vi "Stoplight.vi"() -> ()   [LabVIEW 2023]
uses:
  <vilib>/numeric/Random Number (Range) U64.vi
  <vilib>/numeric/sub_Random U32.vi
panel:
  out "EV Img C":dbl(slide) scale=0.0..10.0
  out "EV img A":dbl(slide) scale=0.0..10.0
  out "EV img b":dbl(slide) scale=0.0..10.0
  out "Car img  C":dbl(slide) scale=0.0..10.0
  out "Car img A":dbl(slide) scale=0.0..10.0
  out "Car img B":dbl(slide) scale=0.0..10.0
  out "EV Alert":bool
  out "EV Changer":dbl
  out "Emergency Lane":bool
  out "stopper":bool
  out "Numeric":i32
  out "EV Num":dbl
  out "Timer":dbl
  in  "Next Lane":string
  out "Indicator":dbl
  in  "Add EV  C":bool
  in  "Add EV  B":bool
  in  "Add EV  A":bool
  in  "Add Ped  C":bool
  in  "Add Ped  B":bool
  in  "Add  Ped A":bool
  in  "Add Car C":bool
  in  "Add Car  B":bool
  in  "Add Car A":bool
  out "Emergency Vehicle C":bool
  out "Emergency Vehicle B":bool
  out "Emergency Vehicle A":bool
  out "Pedestrian C":dbl
  out "Pedestrian B":dbl
  out "Pedestrian A":dbl
  out "Cars C":dbl
  out "Cars B":dbl
  out "Cars A":dbl
  in  "stop":bool
  out "Lane 1g":bool
  out "Lane 3r":bool
  out "Lane 3y":bool
  out "Lane 3g":bool
  out "Lane 2r":bool
  out "Lane 2y":bool
  out "Lane 2g":bool
  out "Lane 1r":bool
  out "Lane 1y":bool
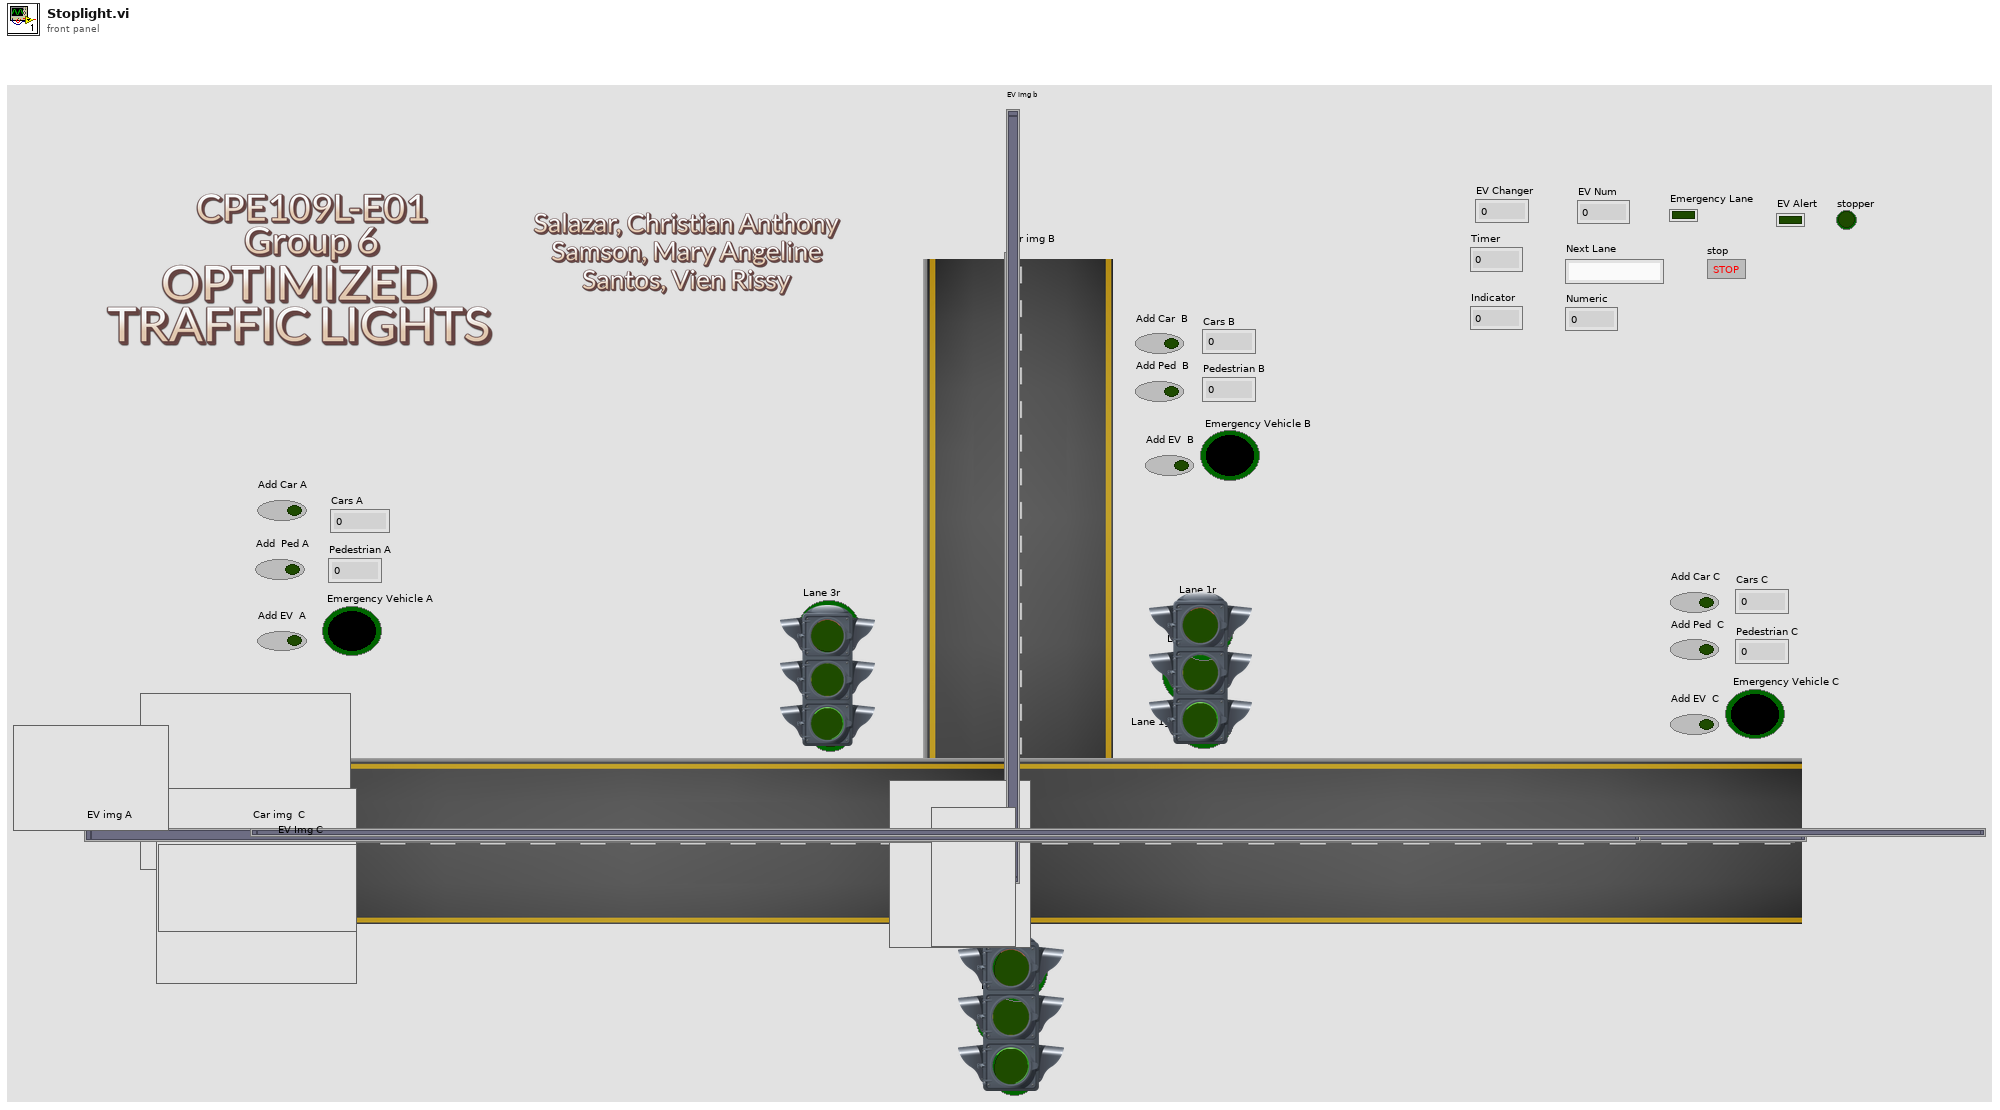
[diagram p1: front panel]
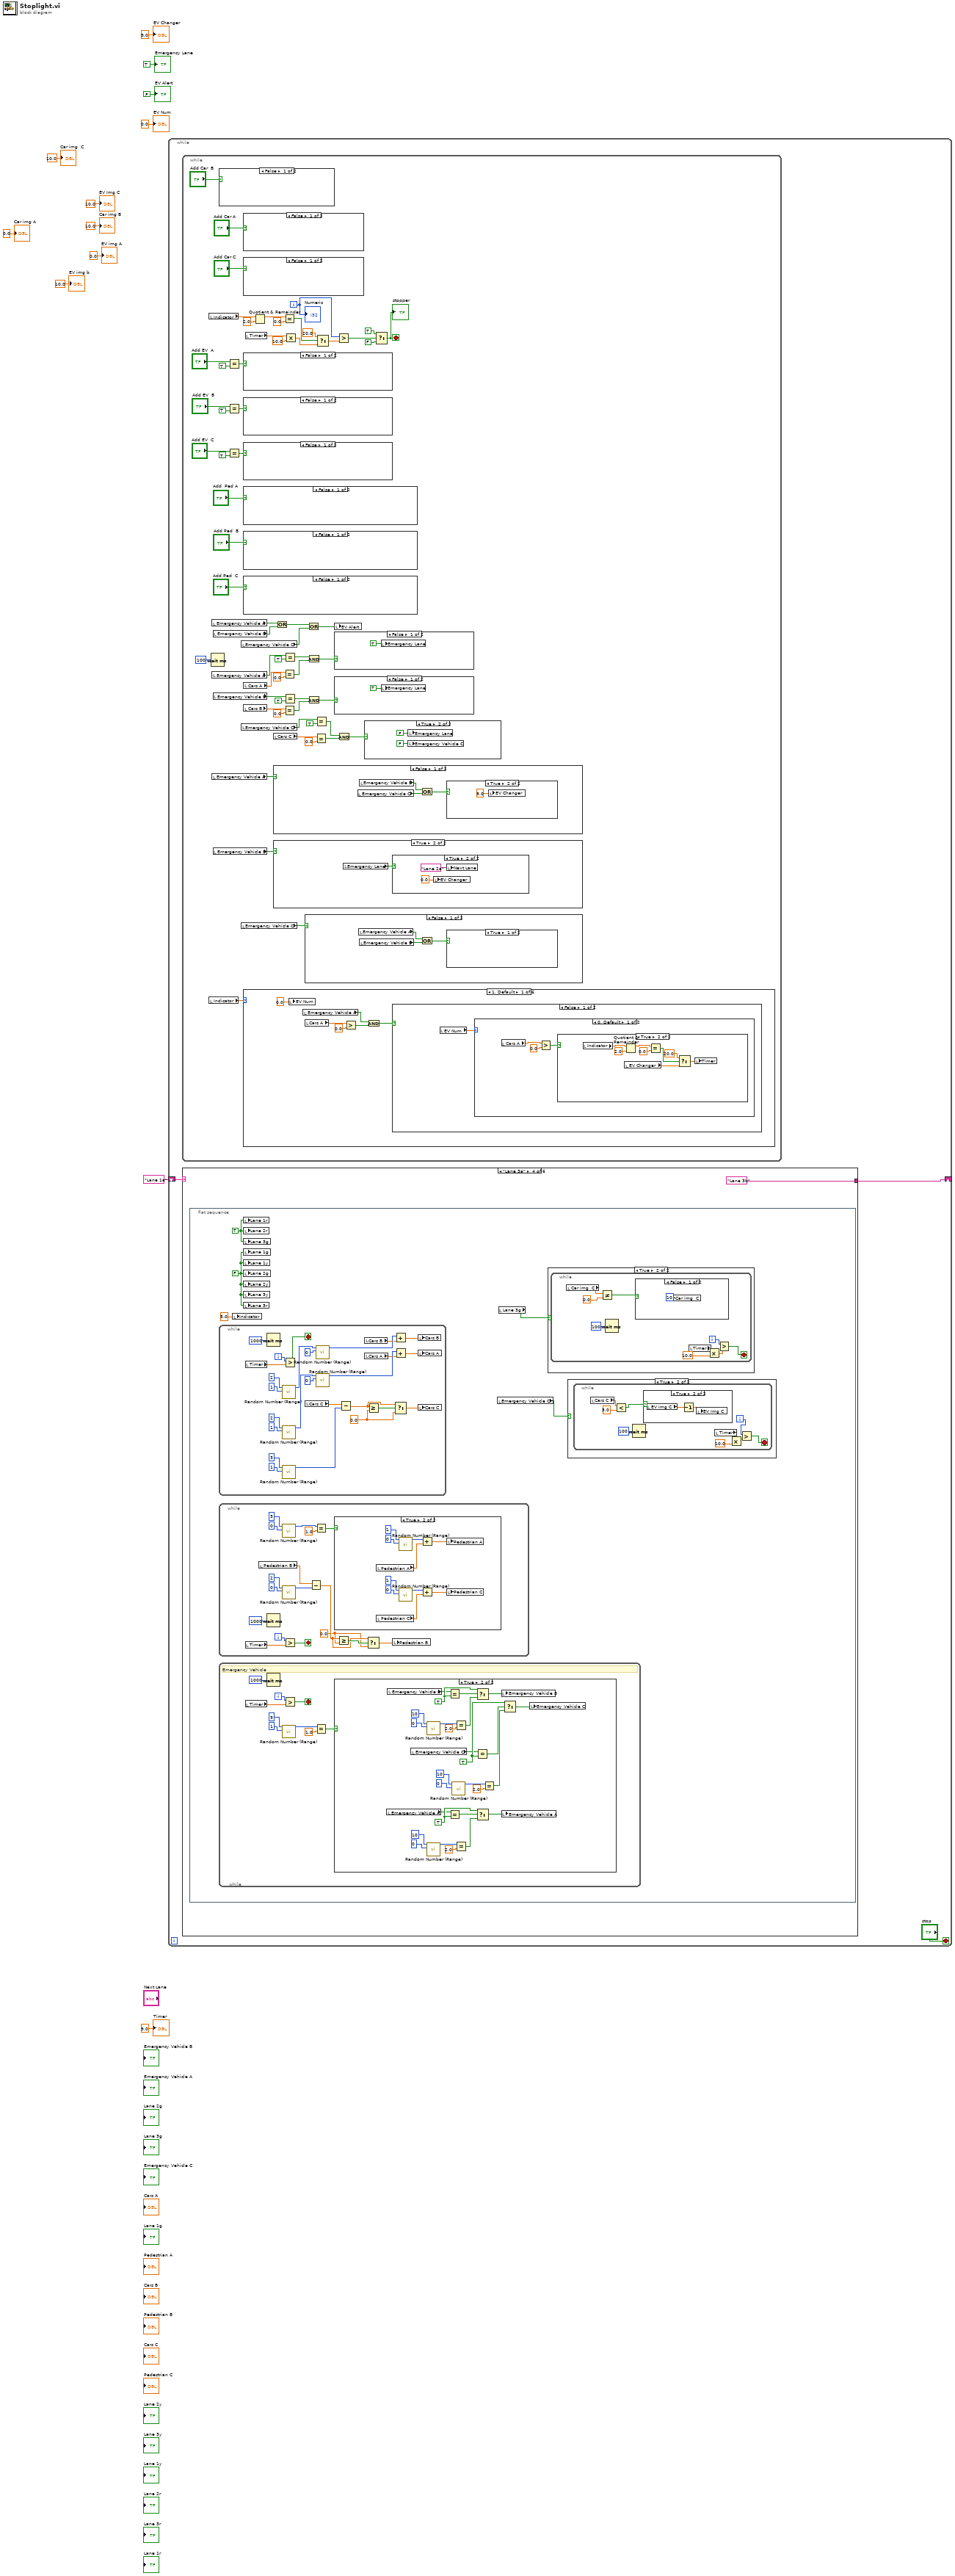
[diagram p0: block diagram]
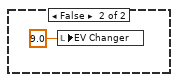
[diagram p2: hidden frame]
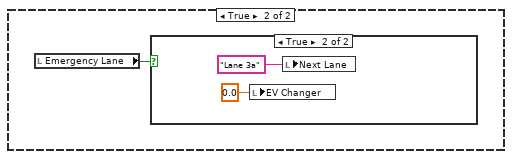
[diagram p3: hidden frame]
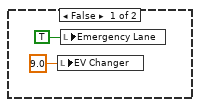
[diagram p4: hidden frame]
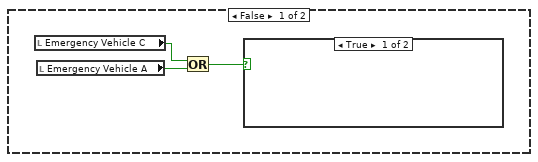
[diagram p5: hidden frame]
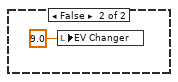
[diagram p6: hidden frame]
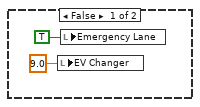
[diagram p7: hidden frame]
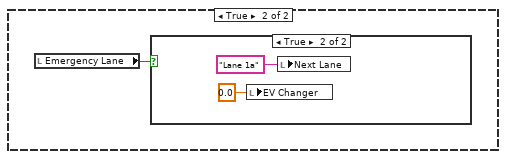
[diagram p9: hidden frame]
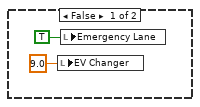
[diagram p10: hidden frame]
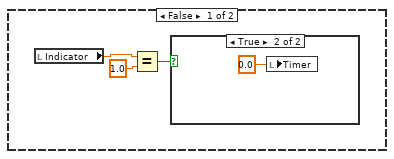
[diagram p11: hidden frame]
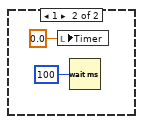
[diagram p13: hidden frame]
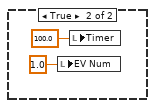
[diagram p14: hidden frame]
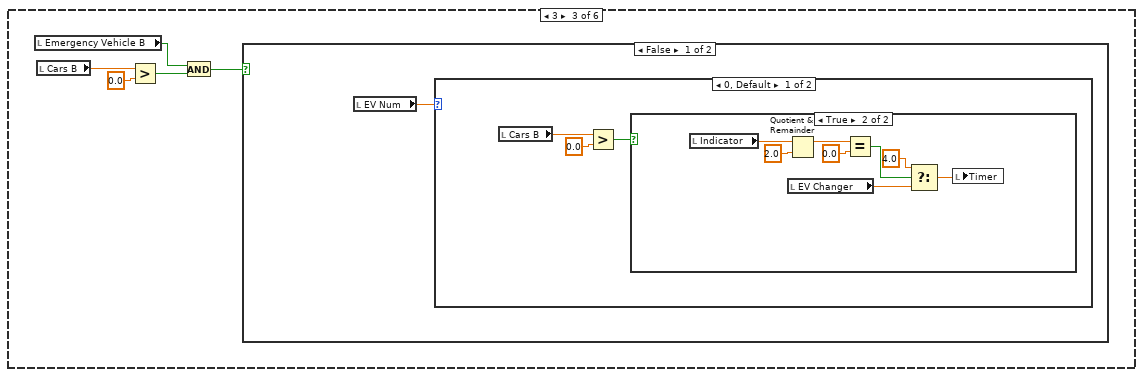
[diagram p16: hidden frame]
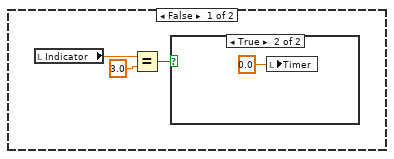
[diagram p17: hidden frame]
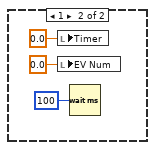
[diagram p19: hidden frame]
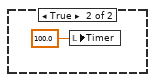
[diagram p20: hidden frame]
diagram:
  n1 = while {
    shift-right: [w13] -> _
    shift-left: "Lane 1a" -> [w14]
    stop <- "stop" stop-if-true
    n2 = while {
      i -> [w34]
      stop <- w73 stop-if-true
      n3 = local read "Indicator"() -> (w58:dbl)
      n4 = local read "Indicator"() -> (w39:dbl)
      n5 = Wait (ms)(milliseconds to wait=u32 100) -> ()  [unwired: 1 out]
      n6 = local read "Emergency Vehicle A"() -> (w20:bool)
      n7 = local read "Emergency Vehicle A"() -> (w45:bool)
      n8 = local read "Emergency Vehicle A"() -> (w32:bool)
      n9 = local read "Emergency Vehicle B"() -> (w19:bool)
      n10 = local read "Emergency Vehicle B"() -> (w43:bool)
      n11 = local read "Emergency Vehicle B"() -> (w31:bool)
      n12 = case shown="False" "Add Car  B" {
        frame False {
        }
        frame True {
          n13 = local read "Cars B"() -> (w201:dbl)
          n14 = Increment(x=w201) -> (x+1=w200:dbl)
          n15 = local write "Cars B"(w200) -> ()
        }
      }
      n16 = Equal?(x="Add EV  A", y=TRUE) -> (x = y?=w61:bool)
      n17 = Equal?(x="Add EV  B", y=TRUE) -> (x = y?=w60:bool)
      n18 = Equal?(x="Add EV  C", y=TRUE) -> (x = y?=w59:bool)
      n19 = local read "Emergency Vehicle C"() -> (w18:bool)
      n20 = local read "Emergency Vehicle C"() -> (w41:bool)
      n21 = local read "Emergency Vehicle C"() -> (w30:bool)
      n22 = case shown="False" "Add Car A" {
        frame False {
        }
        frame True {
          n23 = local read "Cars A"() -> (w203:dbl)
          n24 = Increment(x=w203) -> (x+1=w202:dbl)
          n25 = local write "Cars A"(w202) -> ()
        }
      }
      n26 = case shown="False" "Add Car C" {
        frame False {
        }
        frame True {
          n27 = local read "Cars C"() -> (w199:dbl)
          n28 = Increment(x=w199) -> (x+1=w198:dbl)
          n29 = local write "Cars C"(w198) -> ()
        }
      }
      n30 = case shown="False" w61 {
        frame False {
        }
        frame True {
          n31 = local write "Emergency Vehicle A"(TRUE ("Emergency Vehicle A")) -> ()
        }
      }
      n32 = case shown="False" w60 {
        frame False {
        }
        frame True {
          n33 = local write "Emergency Vehicle B"(TRUE ("Emergency Vehicle B")) -> ()
        }
      }
      n34 = case shown="False" w59 {
        frame False {
        }
        frame True {
          n35 = local write "Emergency Vehicle C"(TRUE ("Emergency Vehicle C")) -> ()
        }
      }
      n36 = case shown="False" "Add  Ped A" {
        frame False {
        }
        frame True {
          n37 = local read "Pedestrian A"() -> (w197:dbl)
          n38 = Increment(x=w197) -> (x+1=w196:dbl)
          n39 = local write "Pedestrian A"(w196) -> ()
        }
      }
      n40 = case shown="False" "Add Ped  B" {
        frame False {
        }
        frame True {
          n41 = local read "Pedestrian B"() -> (w195:dbl)
          n42 = Increment(x=w195) -> (x+1=w194:dbl)
          n43 = local write "Pedestrian B"(w194) -> ()
        }
      }
      n44 = case shown="False" "Add Ped  C" {
        frame False {
        }
        frame True {
          n45 = local read "Pedestrian C"() -> (w193:dbl)
          n46 = Increment(x=w193) -> (x+1=w192:dbl)
          n47 = local write "Pedestrian C"(w192) -> ()
        }
      }
      n48 = local read "Cars A"() -> (w44:dbl)
      n49 = local read "Cars B"() -> (w42:dbl)
      n50 = case shown="1, Default" w39 {
        frame 1, Default {
          n51 = local write "EV Num"(0.0 ("EV Num")) -> ()
          n52 = local read "Emergency Vehicle A"() -> (w107:bool)
          n53 = local read "Cars A"() -> (w108:dbl)
          n54 = Greater?(x=w108, y=0.0) -> (0:w106:bool)
          n55 = And(x=w107, y=w106) -> (x .and. y?=w105:bool)
          n56 = case shown="False" w105 {
            frame False {
              n57 = local read "EV Num"() -> (w110:dbl)
              n58 = case shown="0, Default" w110 {
                frame 0, Default {
                  n59 = local read "Cars A"() -> (w112:dbl)
                  n60 = Greater?(x=w112, y=0.0) -> (0:w113:bool)
                  n61 = case shown="True" w113 {
                    frame False {
                      n62 = local read "Indicator"() -> (w115:dbl)
                      n63 = Equal?(x=w115, y=1.0) -> (x = y?=w114:bool)
                      n64 = case shown="True" w114 {
                        frame False {
                        }
                        frame True {
                          n65 = local write "Timer"(0.0 ("Timer")) -> ()
                        }
                      }
                    }
                    frame True {
                      n66 = local read "Indicator"() -> (w119:dbl)
                      n67 = Quotient & Remainder(x=w119, y=2.0) -> (x-y*floor(x/y)=w123:dbl)  [unwired: 1 out]
                      n68 = local read "EV Changer"() -> (w118:dbl)
                      n69 = Equal?(x=w123, y=0.0) -> (x = y?=w124:bool)
                      n70 = Select(t=20.0, s=w124, f=w118) -> (s? t:f=w120:dbl)
                      n71 = local write "Timer"(w120) -> ()
                    }
                  }
                }
                frame 1 {
                  n72 = local write "Timer"(0.0) -> ()
                  n73 = Wait (ms)(milliseconds to wait=u32 100) -> ()  [unwired: 1 out]
                }
              }
            }
            frame True {
              n74 = local write "EV Num"(1.0 ("EV Num")) -> ()
              n75 = local write "Timer"(100.0) -> ()
            }
          }
        }
        frame 2 {
        }
        frame 3 {
          n76 = local read "Emergency Vehicle B"() -> (w132:bool)
          n77 = local read "Cars B"() -> (w133:dbl)
          n78 = Greater?(x=w133, y=0.0) -> (0:w131:bool)
          n79 = And(x=w132, y=w131) -> (x .and. y?=w130:bool)
          n80 = case shown="False" w130 {
            frame False {
              n81 = local read "EV Num"() -> (w135:dbl)
              n82 = case shown="0, Default" w135 {
                frame 0, Default {
                  n83 = local read "Cars B"() -> (w136:dbl)
                  n84 = Greater?(x=w136, y=0.0) -> (0:w138:bool)
                  n85 = case shown="True" w138 {
                    frame False {
                      n86 = local read "Indicator"() -> (w140:dbl)
                      n87 = Equal?(x=w140, y=3.0) -> (x = y?=w139:bool)
                      n88 = case shown="True" w139 {
                        frame False {
                        }
                        frame True {
                          n89 = local write "Timer"(0.0 ("Timer")) -> ()
                        }
                      }
                    }
                    frame True {
                      n90 = local read "Indicator"() -> (w144:dbl)
                      n91 = Quotient & Remainder(x=w144, y=2.0) -> (x-y*floor(x/y)=w148:dbl)  [unwired: 1 out]
                      n92 = local read "EV Changer"() -> (w143:dbl)
                      n93 = Equal?(x=w148, y=0.0) -> (x = y?=w149:bool)
                      n94 = Select(t=4.0, s=w149, f=w143) -> (s? t:f=w145:dbl)
                      n95 = local write "Timer"(w145) -> ()
                    }
                  }
                }
                frame 1 {
                  n96 = local write "Timer"(0.0) -> ()
                  n97 = local write "EV Num"(0.0) -> ()
                  n98 = Wait (ms)(milliseconds to wait=u32 100) -> ()  [unwired: 1 out]
                }
              }
            }
            frame True {
              n99 = local write "Timer"(100.0) -> ()
            }
          }
        }
        frame 4 {
        }
        frame 5 {
          n100 = local read "Emergency Vehicle C"() -> (w157:bool)
          n101 = local read "Cars C"() -> (w158:dbl)
          n102 = Greater?(x=w158, y=0.0) -> (0:w156:bool)
          n103 = And(x=w157, y=w156) -> (x .and. y?=w155:bool)
          n104 = case shown="False" w155 {
            frame False {
              n105 = local read "EV Num"() -> (w160:dbl)
              n106 = case shown="0, Default" w160 {
                frame 0, Default {
                  n107 = local read "Cars C"() -> (w162:dbl)
                  n108 = Greater?(x=w162, y=0.0) -> (0:w161:bool)
                  n109 = case shown="True" w161 {
                    frame False {
                      n110 = local read "Indicator"() -> (w165:dbl)
                      n111 = Equal?(x=w165, y=5.0) -> (x = y?=w164:bool)
                      n112 = case shown="False" w164 {
                        frame False {
                        }
                        frame True {
                          n113 = local write "Timer"(0.0 ("Timer")) -> ()
                        }
                      }
                    }
                    frame True {
                      n114 = local read "Indicator"() -> (w169:dbl)
                      n115 = Quotient & Remainder(x=w169, y=2.0) -> (x-y*floor(x/y)=w173:dbl)  [unwired: 1 out]
                      n116 = local read "EV Changer"() -> (w168:dbl)
                      n117 = Equal?(x=w173, y=0.0) -> (x = y?=w174:bool)
                      n118 = Select(t=4.0, s=w174, f=w168) -> (s? t:f=w170:dbl)
                      n119 = local write "Timer"(w170) -> ()
                    }
                  }
                }
                frame 1 {
                  n120 = local write "EV Num"(0.0) -> ()
                  n121 = local write "Timer"(0.0) -> ()
                  n122 = Wait (ms)(milliseconds to wait=u32 100) -> ()  [unwired: 1 out]
                }
              }
            }
            frame True {
              n123 = local write "Timer"(100.0) -> ()
            }
          }
        }
        frame 6 {
        }
      }
      n124 = local read "Timer"() -> (w37:dbl)
      n125 = Quotient & Remainder(x=w58, y=2.0) -> (x-y*floor(x/y)=w55:dbl)  [unwired: 1 out]
      n126 = local read "Cars C"() -> (w40:dbl)
      n127 = case shown="False" w32 {
        frame False {
          n128 = local read "Emergency Vehicle C"() -> (w96:bool)
          n129 = local read "Emergency Vehicle B"() -> (w97:bool)
          n130 = Or(x=w97, y=w96) -> (x .or. y?=w95:bool)
          n131 = case shown="True" w95 {
            frame False {
            }
            frame True {
              n132 = local write "EV Changer"(9.0 ("EV Changer")) -> ()
            }
          }
        }
        frame True {
          n133 = local read "Emergency Lane"() -> (w99:bool)
          n134 = case shown="True" w99 {
            frame False {
              n135 = local write "EV Changer"(9.0 ("EV Changer")) -> ()
              n136 = local write "Emergency Lane"(TRUE ("Emergency Lane")) -> ()
            }
            frame True {
              n137 = local write "EV Changer"(0.0 ("Timer")) -> ()
              n138 = local write "Next Lane"("Lane 1a" ("Next Lane")) -> ()
            }
          }
        }
      }
      n139 = case shown="True" w31 {
        frame False {
          n140 = local read "Emergency Vehicle C"() -> (w88:bool)
          n141 = local read "Emergency Vehicle A"() -> (w87:bool)
          n142 = Or(x=w88, y=w87) -> (x .or. y?=w86:bool)
          n143 = case shown="True" w86 {
            frame True {
            }
            frame False {
              n144 = local write "EV Changer"(9.0 ("EV Changer")) -> ()
            }
          }
        }
        frame True {
          n145 = local read "Emergency Lane"() -> (w90:bool)
          n146 = case shown="True" w90 {
            frame False {
              n147 = local write "EV Changer"(9.0 ("EV Changer")) -> ()
              n148 = local write "Emergency Lane"(TRUE ("Emergency Lane")) -> ()
            }
            frame True {
              n149 = local write "EV Changer"(0.0 ("Timer")) -> ()
              n150 = local write "Next Lane"("Lane 2a" ("Next Lane")) -> ()
            }
          }
        }
      }
      n151 = Or(x=w20, y=w19) -> (x .or. y?=w17:bool)
      n152 = Equal?(x=w55, y=0.0) -> (x = y?=w56:bool)
      n153 = Equal?(x=w44, y=0.0) -> (x = y?=w28:bool)
      n154 = Equal?(x=w42, y=0.0) -> (x = y?=w25:bool)
      n155 = Equal?(x=w45, y=TRUE) -> (x = y?=w29:bool)
      n156 = Equal?(x=w43, y=TRUE) -> (x = y?=w26:bool)
      n157 = Multiply(x=w37, y=10.0) -> (x*y=w36:dbl)
      n158 = case shown="False" w30 {
        frame False {
          n159 = local read "Emergency Vehicle A"() -> (w79:bool)
          n160 = local read "Emergency Vehicle B"() -> (w78:bool)
          n161 = Or(x=w79, y=w78) -> (x .or. y?=w77:bool)
          n162 = case shown="True" w77 {
            frame True {
            }
            frame False {
              n163 = local write "EV Changer"(9.0 ("EV Changer")) -> ()
            }
          }
        }
        frame True {
          n164 = local read "Emergency Lane"() -> (w81:bool)
          n165 = case shown="True" w81 {
            frame False {
              n166 = local write "EV Changer"(9.0 ("EV Changer")) -> ()
              n167 = local write "Emergency Lane"(TRUE ("Emergency Lane")) -> ()
            }
            frame True {
              n168 = local write "EV Changer"(0.0 ("Timer")) -> ()
              n169 = local write "Next Lane"("Lane 3a" ("Next Lane")) -> ()
            }
          }
        }
      }
      n170 = Or(x=w17, y=w18) -> (x .or. y?=w16:bool)
      n171 = And(x=w29, y=w28) -> (x .and. y?=w27:bool)
      n172 = And(x=w26, y=w25) -> (x .and. y?=w24:bool)
      n173 = Equal?(x=w40, y=0.0) -> (x = y?=w22:bool)
      n174 = Equal?(x=w41, y=TRUE) -> (x = y?=w23:bool)
      n175 = Select(t=20.0, s=w56, f=w36) -> (s? t:f=w35:dbl)
      n176 = local write "EV Alert"(w16) -> ()
      n177 = case shown="False" w27 {
        frame False {
          n178 = local write "Emergency Lane"(TRUE ("Emergency Lane")) -> ()
        }
        frame True {
          n179 = local write "Emergency Lane"(FALSE) -> ()
          n180 = local write "Emergency Vehicle A"(FALSE) -> ()
        }
      }
      n181 = case shown="False" w24 {
        frame False {
          n182 = local write "Emergency Lane"(TRUE ("Emergency Lane")) -> ()
        }
        frame True {
          n183 = local write "Emergency Lane"(FALSE) -> ()
          n184 = local write "Emergency Vehicle B"(FALSE ("Emergency Vehicle B")) -> ()
        }
      }
      n185 = Greater?(x=w34, y=w35) -> (0:w33:bool)
      n186 = And(x=w23, y=w22) -> (x .and. y?=w21:bool)
      n187 = case shown="True" w21 {
        frame False {
          n188 = local write "Emergency Lane"(TRUE ("Emergency Lane")) -> ()
        }
        frame True {
          n189 = local write "Emergency Lane"(FALSE) -> ()
          n190 = local write "Emergency Vehicle C"(FALSE ("Emergency Vehicle C")) -> ()
        }
      }
      n191 = Select(t=TRUE, s=w33, f=FALSE) -> (s? t:f=w73:bool)
      "stopper" <- w73
      "Numeric" <- w34
    }
    n192 = case shown="\"Lane 3a\"" w14 {
      tunnel: [w207 "Lane 2b" w334 "Lane 3b" w470 "Lane 1b"] -> w13
      frame "Lane 1b" {
        n193 = flat-sequence {
          frame #0 {
            w217 = FALSE
            w218 = TRUE
            n194 = local write "Timer"(4.0 ("Timer")) -> ()
            n195 = local write "Indicator"(2.0 ("Indicator")) -> ()
            n196 = Wait (ms)(milliseconds to wait=u32 2000) -> ()  [unwired: 1 out]
            n197 = local write "Lane 1g"(w217) -> ()
            n198 = local write "Lane 1r"(w217) -> ()
            n199 = local write "Lane 2g"(w217) -> ()
            n200 = local write "Lane 2y"(w217) -> ()
            n201 = local write "Lane 3g"(w217) -> ()
            n202 = local write "Lane 3y"(w217) -> ()
            n203 = local write "Lane 1y"(w218) -> ()
            n204 = local write "Lane 2r"(w218) -> ()
            n205 = local write "Lane 3r"(w218) -> ()
            n206 = local write "Car img B"(10) -> ()
            n207 = local write "EV img A"(0) -> ()
            n208 = local write "Car img  C"(10) -> ()
            n209 = local write "EV Img C"(10) -> ()
            n210 = local write "EV img b"(10) -> ()
            n211 = local write "Car img A"(0) -> ()
          }
        }
        n212 = local read "Next Lane"() -> (w204:string)
        n213 = local read "EV Alert"() -> (w206:bool)
        n214 = Select(t=w204, s=w206, f="Lane 2a") -> (s? t:f=w207:string)
      }
      frame "Lane 2a" {
        n215 = flat-sequence {
          frame #0 {
            w223 = FALSE
            w224 = TRUE
            n216 = while {
              stop <- w310 stop-if-true
              w322 = 0.0 ("y")
              # "Cars"
              n217 = Wait (ms)(milliseconds to wait=u32 1000) -> ()  [unwired: 1 out]
              n218 = call-poly <vilib>:"Random Number (Range).vi"("lower bound (0)"=u64 1, "upper bound (100)"=u64 2) -> ("number"=w311:u64)  [unwired: 9 in]
              n219 = call-poly <vilib>:"Random Number (Range).vi"("lower bound (0)"=u64 1, "upper bound (100)"=u64 2) -> ("number"=w314:u64)  [unwired: 9 in]
              n220 = call-poly <vilib>:"Random Number (Range).vi"("lower bound (0)"=u64 1, "upper bound (100)"=u64 3) -> ("number"=w317:u64)  [unwired: 9 in]
              n221 = local read "Cars B"() -> (w321:dbl)
              n222 = call-poly <vilib>:"Random Number (Range).vi"("lower bound (0)"=u64 0, "upper bound (100)"=w311) -> ("number"=w326:u64)  [unwired: 9 in]
              n223 = call-poly <vilib>:"Random Number (Range).vi"("lower bound (0)"=u64 0, "upper bound (100)"=w314) -> ("number"=w328:u64)  [unwired: 9 in]
              n224 = Subtract(x=w321, y=w317) -> (x-y=w323:dbl)
              n225 = local read "Cars C"() -> (w329:dbl)
              n226 = local read "Cars A"() -> (w330:dbl)
              n227 = Greater Or Equal?(x=w323, y=w322) -> (x >= y?=w324:bool)
              n228 = Add(x=w326, y=w329) -> (x+y=w325:dbl)
              n229 = Add(x=w328, y=w330) -> (x+y=w327:dbl)
              n230 = Select(t=w323, s=w324, f=w322) -> (s? t:f=w320:dbl)
              n231 = local read "stopper"() -> (w310:bool)
              n232 = local write "Cars C"(w325) -> ()
              n233 = local write "Cars A"(w327) -> ()
              n234 = local write "Cars B"(w320) -> ()
            }
            n235 = while {
              stop <- w285 stop-if-true
              w290 = 0.0 ("y")
              # "Pedestrian"
              n236 = local read "Pedestrian A"() -> (w293:dbl)
              n237 = Wait (ms)(milliseconds to wait=u32 1000) -> ()  [unwired: 1 out]
              n238 = call-poly <vilib>:"Random Number (Range).vi"("lower bound (0)"=u64 0, "upper bound (100)"=u64 3) -> ("number"=w295:u64)  [unwired: 9 in]
              n239 = call-poly <vilib>:"Random Number (Range).vi"("lower bound (0)"=u64 0, "upper bound (100)"=u64 2) -> ("number"=w286:u64)  [unwired: 9 in]
              n240 = Subtract(x=w293, y=w286) -> (x-y=w291:dbl)
              n241 = Equal?(x=w295, y=1.0) -> (x = y?=w294:bool)
              n242 = case shown="False" w294 {
                frame False {
                }
                frame True {
                  n243 = local read "Pedestrian B"() -> (w303:dbl)
                  n244 = local read "Pedestrian C"() -> (w301:dbl)
                  n245 = call-poly <vilib>:"Random Number (Range).vi"("lower bound (0)"=u64 0, "upper bound (100)"=u64 1) -> ("number"=w305:u64)  [unwired: 9 in]
                  n246 = call-poly <vilib>:"Random Number (Range).vi"("lower bound (0)"=u64 0, "upper bound (100)"=u64 1) -> ("number"=w304:u64)  [unwired: 9 in]
                  n247 = Add(x=w305, y=w303) -> (x+y=w302:dbl)
                  n248 = Add(x=w304, y=w301) -> (x+y=w300:dbl)
                  n249 = local write "Pedestrian B"(w302) -> ()
                  n250 = local write "Pedestrian C"(w300) -> ()
                }
              }
              n251 = Greater Or Equal?(x=w291, y=w290) -> (x >= y?=w292:bool)
              n252 = Select(t=w291, s=w292, f=w290) -> (s? t:f=w289:dbl)
              n253 = local write "Pedestrian A"(w289) -> ()
              n254 = local read "stopper"() -> (w285:bool)
            }
            n255 = while {
              stop <- w251 stop-if-true
              # "Emergency Vehicle"
              n256 = Wait (ms)(milliseconds to wait=u32 1000) -> ()  [unwired: 1 out]
              n257 = call-poly <vilib>:"Random Number (Range).vi"("lower bound (0)"=u64 1, "upper bound (100)"=u64 25) -> ("number"=w252:u64)  [unwired: 9 in]
              n258 = Equal?(x=w252, y=1.0) -> (x = y?=w254:bool)
              n259 = case shown="False" w254 {
                frame False {
                }
                frame True {
                  w266 = TRUE
                  w265 = TRUE
                  w264 = TRUE
                  n260 = local read "Emergency Vehicle A"() -> (w260:bool)
                  n261 = local read "Emergency Vehicle B"() -> (w259:bool)
                  n262 = local read "Emergency Vehicle C"() -> (w258:bool)
                  n263 = call-poly <vilib>:"Random Number (Range).vi"("lower bound (0)"=u64 0, "upper bound (100)"=u64 10) -> ("number"=w274:u64)  [unwired: 9 in]
                  n264 = call-poly <vilib>:"Random Number (Range).vi"("lower bound (0)"=u64 0, "upper bound (100)"=u64 10) -> ("number"=w275:u64)  [unwired: 9 in]
                  n265 = Equal?(x=w259, y=w265) -> (x = y?=w268:bool)
                  n266 = Equal?(x=w260, y=w264) -> (x = y?=w269:bool)
                  n267 = call-poly <vilib>:"Random Number (Range).vi"("lower bound (0)"=u64 0, "upper bound (100)"=u64 10) -> ("number"=w273:u64)  [unwired: 9 in]
                  n268 = Equal?(x=w274, y=2.0) -> (x = y?=w262:bool)
                  n269 = Equal?(x=w275, y=2.0) -> (x = y?=w263:bool)
                  n270 = Select(t=w265, s=w268, f=w262) -> (s? t:f=w271:bool)
                  n271 = Equal?(x=w258, y=w266) -> (x = y?=w267:bool)
                  n272 = Select(t=w264, s=w269, f=w263) -> (s? t:f=w272:bool)
                  n273 = Equal?(x=w273, y=2.0) -> (x = y?=w261:bool)
                  n274 = local write "Emergency Vehicle B"(w271) -> ()
                  n275 = local write "Emergency Vehicle A"(w272) -> ()
                  n276 = Select(t=w266, s=w267, f=w261) -> (s? t:f=w270:bool)
                  n277 = local write "Emergency Vehicle C"(w270) -> ()
                }
              }
              n278 = local read "stopper"() -> (w251:bool)
            }
            n279 = local write "Indicator"(3.0 ("Indicator")) -> ()
            n280 = local write "Lane 1r"(w224) -> ()
            n281 = local write "Lane 2g"(w224) -> ()
            n282 = local write "Lane 3r"(w224) -> ()
            n283 = local write "Lane 1g"(w223) -> ()
            n284 = local write "Lane 1y"(w223) -> ()
            n285 = local write "Lane 2y"(w223) -> ()
            n286 = local write "Lane 2r"(w223) -> ()
            n287 = local write "Lane 3g"(w223) -> ()
            n288 = local write "Lane 3y"(w223) -> ()
            n289 = local read "Emergency Vehicle B"() -> (w220:bool)
            n290 = local read "Lane 2g"() -> (w221:bool)
            n291 = case shown="True" w221 {
              frame False {
                n292 = local write "Car img B"(10.0 ("Car img B")) -> ()
              }
              frame True {
                n293 = while {
                  i -> [w246]
                  stop <- w243 stop-if-true
                  n294 = local read "Car img B"() -> (w241:dbl)
                  n295 = Wait (ms)(milliseconds to wait=u32 100) -> ()  [unwired: 1 out]
                  n296 = Greater?(x=w241, y=1.0) -> (0:w239:bool)
                  n297 = case shown="True" w239 {
                    frame False {
                      n298 = local write "Car img B"(10.0 ("Car img B")) -> ()
                    }
                    frame True {
                      n299 = local read "Car img B"() -> (w250:dbl)
                      n300 = Decrement(x=w250) -> (x-1=w249:dbl)
                      n301 = local write "Car img B"(w249) -> ()
                    }
                  }
                  n302 = local read "Timer"() -> (w245:dbl)
                  n303 = Multiply(x=w245, y=10.0) -> (x*y=w242:dbl)
                  n304 = Greater?(x=w246, y=w242) -> (0:w243:bool)
                }
              }
            }
            n305 = case shown="True" w220 {
              frame False {
                n306 = local write "EV img b"(10.0 ("EV img b")) -> ()
              }
              frame True {
                n307 = while {
                  i -> [w229]
                  stop <- w227 stop-if-true
                  n308 = local read "Cars B"() -> (w233:dbl)
                  n309 = Less?(x=w233, y=5.0) -> (x < y?=w232:bool)
                  n310 = Wait (ms)(milliseconds to wait=u32 100) -> ()  [unwired: 1 out]
                  n311 = case shown="True" w232 {
                    frame False {
                      n312 = local write "EV img b"(10) -> ()
                    }
                    frame True {
                      n313 = local read "EV img b"() -> (w237:dbl)
                      n314 = Decrement(x=w237) -> (x-1=w236:dbl)
                      n315 = local write "EV img b"(w236) -> ()
                    }
                  }
                  n316 = local read "Timer"() -> (w231:dbl)
                  n317 = Multiply(x=w231, y=10.0) -> (x*y=w228:dbl)
                  n318 = Greater?(x=w229, y=w228) -> (0:w227:bool)
                }
              }
            }
          }
        }
      }
      frame "Lane 2b" {
        n319 = flat-sequence {
          frame #0 {
            w346 = FALSE
            w347 = TRUE
            n320 = local write "Timer"(4.0 ("Timer")) -> ()
            n321 = local write "Indicator"(4.0 ("Indicator")) -> ()
            n322 = Wait (ms)(milliseconds to wait=u32 2000) -> ()  [unwired: 1 out]
            n323 = local write "Lane 1g"(w346) -> ()
            n324 = local write "Lane 1y"(w346) -> ()
            n325 = local write "Lane 2g"(w346) -> ()
            n326 = local write "Lane 2r"(w346) -> ()
            n327 = local write "Lane 3g"(w346) -> ()
            n328 = local write "Lane 3y"(w346) -> ()
            n329 = local write "Lane 1r"(w347) -> ()
            n330 = local write "Lane 2y"(w347) -> ()
            n331 = local write "Lane 3r"(w347) -> ()
            n332 = local write "EV Img C"(10) -> ()
            n333 = local write "Car img  C"(10) -> ()
            n334 = local write "EV img A"(0) -> ()
            n335 = local write "Car img B"(10) -> ()
            n336 = local write "EV img b"(10) -> ()
            n337 = local write "Car img A"(0) -> ()
          }
        }
        n338 = local read "Next Lane"() -> (w336:string)
        n339 = local read "EV Alert"() -> (w337:bool)
        n340 = Select(t=w336, s=w337, f="Lane 3a") -> (s? t:f=w334:string)
      }
      frame "Lane 3a" {
        n341 = flat-sequence {
          frame #0 {
            w353 = FALSE
            w354 = TRUE
            n342 = while {
              i -> [w452]
              stop <- w451 stop-if-true
              w458 = 0.0 ("y")
              n343 = local read "Timer"() -> (w450:dbl)
              n344 = Wait (ms)(milliseconds to wait=u32 1000) -> ()  [unwired: 1 out]
              n345 = call-poly <vilib>:"Random Number (Range).vi"("lower bound (0)"=u64 1, "upper bound (100)"=u64 2) -> ("number"=w444:u64)  [unwired: 9 in]
              n346 = call-poly <vilib>:"Random Number (Range).vi"("lower bound (0)"=u64 1, "upper bound (100)"=u64 2) -> ("number"=w447:u64)  [unwired: 9 in]
              n347 = call-poly <vilib>:"Random Number (Range).vi"("lower bound (0)"=u64 1, "upper bound (100)"=u64 3) -> ("number"=w453:u64)  [unwired: 9 in]
              n348 = Greater?(x=w452, y=w450) -> (0:w451:bool)
              n349 = local read "Cars C"() -> (w457:dbl)
              n350 = call-poly <vilib>:"Random Number (Range).vi"("lower bound (0)"=u64 0, "upper bound (100)"=w444) -> ("number"=w463:u64)  [unwired: 9 in]
              n351 = call-poly <vilib>:"Random Number (Range).vi"("lower bound (0)"=u64 0, "upper bound (100)"=w447) -> ("number"=w466:u64)  [unwired: 9 in]
              n352 = Subtract(x=w457, y=w453) -> (x-y=w459:dbl)
              n353 = local read "Cars B"() -> (w462:dbl)
              n354 = local read "Cars A"() -> (w465:dbl)
              n355 = Greater Or Equal?(x=w459, y=w458) -> (x >= y?=w460:bool)
              n356 = Add(x=w463, y=w462) -> (x+y=w461:dbl)
              n357 = Add(x=w466, y=w465) -> (x+y=w464:dbl)
              n358 = Select(t=w459, s=w460, f=w458) -> (s? t:f=w456:dbl)
              n359 = local write "Cars B"(w461) -> ()
              n360 = local write "Cars A"(w464) -> ()
              n361 = local write "Cars C"(w456) -> ()
            }
            n362 = while {
              i -> [w419]
              stop <- w418 stop-if-true
              w423 = 0.0 ("y")
              n363 = local read "Timer"() -> (w417:dbl)
              n364 = local read "Pedestrian B"() -> (w427:dbl)
              n365 = Wait (ms)(milliseconds to wait=u32 1000) -> ()  [unwired: 1 out]
              n366 = call-poly <vilib>:"Random Number (Range).vi"("lower bound (0)"=u64 0, "upper bound (100)"=u64 3) -> ("number"=w429:u64)  [unwired: 9 in]
              n367 = call-poly <vilib>:"Random Number (Range).vi"("lower bound (0)"=u64 0, "upper bound (100)"=u64 2) -> ("number"=w420:u64)  [unwired: 9 in]
              n368 = Greater?(x=w419, y=w417) -> (0:w418:bool)
              n369 = Subtract(x=w427, y=w420) -> (x-y=w424:dbl)
              n370 = Equal?(x=w429, y=1.0) -> (x = y?=w428:bool)
              n371 = case shown="True" w428 {
                frame False {
                }
                frame True {
                  n372 = local read "Pedestrian A"() -> (w437:dbl)
                  n373 = local read "Pedestrian C"() -> (w435:dbl)
                  n374 = call-poly <vilib>:"Random Number (Range).vi"("lower bound (0)"=u64 0, "upper bound (100)"=u64 1) -> ("number"=w439:u64)  [unwired: 9 in]
                  n375 = call-poly <vilib>:"Random Number (Range).vi"("lower bound (0)"=u64 0, "upper bound (100)"=u64 1) -> ("number"=w438:u64)  [unwired: 9 in]
                  n376 = Add(x=w439, y=w437) -> (x+y=w436:dbl)
                  n377 = Add(x=w438, y=w435) -> (x+y=w434:dbl)
                  n378 = local write "Pedestrian A"(w436) -> ()
                  n379 = local write "Pedestrian C"(w434) -> ()
                }
              }
              n380 = Greater Or Equal?(x=w424, y=w423) -> (x >= y?=w425:bool)
              n381 = Select(t=w424, s=w425, f=w423) -> (s? t:f=w426:dbl)
              n382 = local write "Pedestrian B"(w426) -> ()
            }
            n383 = while {
              i -> [w383]
              stop <- w382 stop-if-true
              # "Emergency Vehicle"
              n384 = local read "Timer"() -> (w381:dbl)
              n385 = Wait (ms)(milliseconds to wait=u32 1000) -> ()  [unwired: 1 out]
              n386 = call-poly <vilib>:"Random Number (Range).vi"("lower bound (0)"=u64 1, "upper bound (100)"=u64 9) -> ("number"=w384:u64)  [unwired: 9 in]
              n387 = Greater?(x=w383, y=w381) -> (0:w382:bool)
              n388 = Equal?(x=w384, y=1.0) -> (x = y?=w386:bool)
              n389 = case shown="True" w386 {
                frame False {
                }
                frame True {
                  w401 = TRUE
                  w400 = TRUE
                  w399 = TRUE
                  n390 = local read "Emergency Vehicle A"() -> (w392:bool)
                  n391 = local read "Emergency Vehicle B"() -> (w391:bool)
                  n392 = local read "Emergency Vehicle C"() -> (w390:bool)
                  n393 = call-poly <vilib>:"Random Number (Range).vi"("lower bound (0)"=u64 0, "upper bound (100)"=u64 10) -> ("number"=w406:u64)  [unwired: 9 in]
                  n394 = call-poly <vilib>:"Random Number (Range).vi"("lower bound (0)"=u64 0, "upper bound (100)"=u64 10) -> ("number"=w407:u64)  [unwired: 9 in]
                  n395 = Equal?(x=w391, y=w400) -> (x = y?=w403:bool)
                  n396 = Equal?(x=w392, y=w399) -> (x = y?=w404:bool)
                  n397 = call-poly <vilib>:"Random Number (Range).vi"("lower bound (0)"=u64 0, "upper bound (100)"=u64 10) -> ("number"=w405:u64)  [unwired: 9 in]
                  n398 = Equal?(x=w406, y=2.0) -> (x = y?=w397:bool)
                  n399 = Equal?(x=w407, y=2.0) -> (x = y?=w398:bool)
                  n400 = Select(t=w400, s=w403, f=w397) -> (s? t:f=w394:bool)
                  n401 = Equal?(x=w390, y=w401) -> (x = y?=w402:bool)
                  n402 = Select(t=w399, s=w404, f=w398) -> (s? t:f=w395:bool)
                  n403 = Equal?(x=w405, y=2.0) -> (x = y?=w396:bool)
                  n404 = local write "Emergency Vehicle B"(w394) -> ()
                  n405 = local write "Emergency Vehicle A"(w395) -> ()
                  n406 = Select(t=w401, s=w402, f=w396) -> (s? t:f=w393:bool)
                  n407 = local write "Emergency Vehicle C"(w393) -> ()
                }
              }
            }
            n408 = local write "Indicator"(5.0 ("Indicator")) -> ()
            n409 = local write "Lane 1r"(w354) -> ()
            n410 = local write "Lane 2r"(w354) -> ()
            n411 = local write "Lane 3g"(w354) -> ()
            n412 = local write "Lane 1g"(w353) -> ()
            n413 = local write "Lane 1y"(w353) -> ()
            n414 = local write "Lane 2g"(w353) -> ()
            n415 = local write "Lane 2y"(w353) -> ()
            n416 = local write "Lane 3y"(w353) -> ()
            n417 = local write "Lane 3r"(w353) -> ()
            n418 = local read "Emergency Vehicle C"() -> (w350:bool)
            n419 = local read "Lane 3g"() -> (w351:bool)
            n420 = case shown="True" w351 {
              frame False {
                n421 = local write "Car img  C"(10.0 ("Car img  C")) -> ()
              }
              frame True {
                n422 = while {
                  i -> [w373]
                  stop <- w369 stop-if-true
                  n423 = local read "Car img  C"() -> (w376:dbl)
                  n424 = Not Equal?(x=w376, y=0.0) -> (x != y?=w375:bool)
                  n425 = Wait (ms)(milliseconds to wait=u32 100) -> ()  [unwired: 1 out]
                  n426 = case shown="False" w375 {
                    frame False {
                      n427 = local write "Car img  C"(10) -> ()
                    }
                    frame True {
                      n428 = local read "Car img  C"() -> (w380:dbl)
                      n429 = Decrement(x=w380) -> (x-1=w379:dbl)
                      n430 = local write "Car img  C"(w379) -> ()
                    }
                  }
                  n431 = local read "Timer"() -> (w372:dbl)
                  n432 = Multiply(x=w372, y=10.0) -> (x*y=w370:dbl)
                  n433 = Greater?(x=w373, y=w370) -> (0:w369:bool)
                }
              }
            }
            n434 = case shown="True" w350 {
              frame False {
                n435 = local write "EV Img C"(10.0 ("EV Img C")) -> ()
              }
              frame True {
                n436 = while {
                  i -> [w359]
                  stop <- w357 stop-if-true
                  n437 = local read "Cars C"() -> (w363:dbl)
                  n438 = Less?(x=w363, y=5.0) -> (x < y?=w362:bool)
                  n439 = Wait (ms)(milliseconds to wait=u32 100) -> ()  [unwired: 1 out]
                  n440 = case shown="True" w362 {
                    frame False {
                      n441 = local write "EV Img C"(10) -> ()
                    }
                    frame True {
                      n442 = local read "EV Img C"() -> (w367:dbl)
                      n443 = Decrement(x=w367) -> (x-1=w366:dbl)
                      n444 = local write "EV Img C"(w366) -> ()
                    }
                  }
                  n445 = local read "Timer"() -> (w361:dbl)
                  n446 = Multiply(x=w361, y=10.0) -> (x*y=w358:dbl)
                  n447 = Greater?(x=w359, y=w358) -> (0:w357:bool)
                }
              }
            }
          }
        }
      }
      frame "Lane 3b" {
        n448 = flat-sequence {
          frame #0 {
            w482 = FALSE
            w483 = TRUE
            n449 = local write "Timer"(4.0 ("Timer")) -> ()
            n450 = local write "Indicator"(6.0 ("Indicator")) -> ()
            n451 = Wait (ms)(milliseconds to wait=u32 2000) -> ()  [unwired: 1 out]
            n452 = local write "Lane 1g"(w482) -> ()
            n453 = local write "Lane 1y"(w482) -> ()
            n454 = local write "Lane 2g"(w482) -> ()
            n455 = local write "Lane 2y"(w482) -> ()
            n456 = local write "Lane 3g"(w482) -> ()
            n457 = local write "Lane 3r"(w482) -> ()
            n458 = local write "Lane 1r"(w483) -> ()
            n459 = local write "Lane 2r"(w483) -> ()
            n460 = local write "Lane 3y"(w483) -> ()
            n461 = local write "EV Img C"(10) -> ()
            n462 = local write "Car img  C"(10) -> ()
            n463 = local write "EV img A"(0) -> ()
            n464 = local write "Car img B"(10) -> ()
            n465 = local write "EV img b"(10) -> ()
            n466 = local write "Car img A"(0) -> ()
          }
        }
        n467 = local read "Next Lane"() -> (w472:string)
        n468 = local read "EV Alert"() -> (w473:bool)
        n469 = Select(t=w472, s=w473, f="Lane 1a") -> (s? t:f=w470:string)
      }
      frame "Lane 1a", Default {
        n470 = flat-sequence {
          frame #0 {
            w489 = FALSE
            w490 = TRUE
            n471 = while {
              i -> [w587]
              stop <- w588 stop-if-true
              w595 = 0.0 ("y")
              n472 = local read "Timer"() -> (w586:dbl)
              n473 = Wait (ms)(milliseconds to wait=u32 1000) -> ()  [unwired: 1 out]
              n474 = call-poly <vilib>:"Random Number (Range).vi"("lower bound (0)"=u64 1, "upper bound (100)"=u64 2) -> ("number"=w580:u64)  [unwired: 9 in]
              n475 = call-poly <vilib>:"Random Number (Range).vi"("lower bound (0)"=u64 1, "upper bound (100)"=u64 2) -> ("number"=w583:u64)  [unwired: 9 in]
              n476 = call-poly <vilib>:"Random Number (Range).vi"("lower bound (0)"=u64 1, "upper bound (100)"=u64 3) -> ("number"=w589:u64)  [unwired: 9 in]
              n477 = Greater?(x=w587, y=w586) -> (0:w588:bool)
              n478 = local read "Cars A"() -> (w594:dbl)
              n479 = call-poly <vilib>:"Random Number (Range).vi"("lower bound (0)"=u64 0, "upper bound (100)"=w580) -> ("number"=w601:u64)  [unwired: 9 in]
              n480 = call-poly <vilib>:"Random Number (Range).vi"("lower bound (0)"=u64 0, "upper bound (100)"=w583) -> ("number"=w603:u64)  [unwired: 9 in]
              n481 = Subtract(x=w594, y=w589) -> (x-y=w596:dbl)
              n482 = local read "Cars C"() -> (w600:dbl)
              n483 = local read "Cars B"() -> (w602:dbl)
              n484 = Greater Or Equal?(x=w596, y=w595) -> (x >= y?=w597:bool)
              n485 = Add(x=w601, y=w600) -> (x+y=w599:dbl)
              n486 = Add(x=w603, y=w602) -> (x+y=w598:dbl)
              n487 = Select(t=w596, s=w597, f=w595) -> (s? t:f=w593:dbl)
              n488 = local write "Cars C"(w599) -> ()
              n489 = local write "Cars B"(w598) -> ()
              n490 = local write "Cars A"(w593) -> ()
            }
            n491 = while {
              i -> [w555]
              stop <- w554 stop-if-true
              w567 = 0.0 ("y")
              n492 = local read "Timer"() -> (w553:dbl)
              n493 = local read "Pedestrian C"() -> (w560:dbl)
              n494 = Wait (ms)(milliseconds to wait=u32 1000) -> ()  [unwired: 1 out]
              n495 = call-poly <vilib>:"Random Number (Range).vi"("lower bound (0)"=u64 0, "upper bound (100)"=u64 2) -> ("number"=w556:u64)  [unwired: 9 in]
              n496 = call-poly <vilib>:"Random Number (Range).vi"("lower bound (0)"=u64 0, "upper bound (100)"=u64 3) -> ("number"=w561:u64)  [unwired: 9 in]
              n497 = Greater?(x=w555, y=w553) -> (0:w554:bool)
              n498 = Subtract(x=w560, y=w556) -> (x-y=w559:dbl)
              n499 = Equal?(x=w561, y=1.0) -> (x = y?=w564:bool)
              n500 = case shown="True" w564 {
                frame False {
                }
                frame True {
                  n501 = local read "Pedestrian B"() -> (w572:dbl)
                  n502 = local read "Pedestrian A"() -> (w574:dbl)
                  n503 = call-poly <vilib>:"Random Number (Range).vi"("lower bound (0)"=u64 0, "upper bound (100)"=u64 1) -> ("number"=w575:u64)  [unwired: 9 in]
                  n504 = call-poly <vilib>:"Random Number (Range).vi"("lower bound (0)"=u64 0, "upper bound (100)"=u64 1) -> ("number"=w571:u64)  [unwired: 9 in]
                  n505 = Add(x=w575, y=w574) -> (x+y=w573:dbl)
                  n506 = Add(x=w571, y=w572) -> (x+y=w570:dbl)
                  n507 = local write "Pedestrian A"(w573) -> ()
                  n508 = local write "Pedestrian B"(w570) -> ()
                }
              }
              n509 = Greater Or Equal?(x=w559, y=w567) -> (x >= y?=w568:bool)
              n510 = Select(t=w559, s=w568, f=w567) -> (s? t:f=w566:dbl)
              n511 = local write "Pedestrian C"(w566) -> ()
            }
            n512 = while {
              i -> [w518]
              stop <- w519 stop-if-true
              # "Emergency Vehicle"
              n513 = local read "Timer"() -> (w517:dbl)
              n514 = Wait (ms)(milliseconds to wait=u32 1000) -> ()  [unwired: 1 out]
              n515 = call-poly <vilib>:"Random Number (Range).vi"("lower bound (0)"=u64 0, "upper bound (100)"=u64 25) -> ("number"=w520:u64)  [unwired: 9 in]
              n516 = Greater?(x=w518, y=w517) -> (0:w519:bool)
              n517 = Equal?(x=w520, y=1.0) -> (x = y?=w522:bool)
              n518 = case shown="False" w522 {
                frame False {
                }
                frame True {
                  w537 = TRUE
                  w536 = TRUE
                  w535 = TRUE
                  n519 = local read "Emergency Vehicle A"() -> (w528:bool)
                  n520 = local read "Emergency Vehicle B"() -> (w527:bool)
                  n521 = local read "Emergency Vehicle C"() -> (w526:bool)
                  n522 = call-poly <vilib>:"Random Number (Range).vi"("lower bound (0)"=u64 0, "upper bound (100)"=u64 10) -> ("number"=w542:u64)  [unwired: 9 in]
                  n523 = call-poly <vilib>:"Random Number (Range).vi"("lower bound (0)"=u64 0, "upper bound (100)"=u64 10) -> ("number"=w543:u64)  [unwired: 9 in]
                  n524 = Equal?(x=w527, y=w536) -> (x = y?=w539:bool)
                  n525 = Equal?(x=w528, y=w535) -> (x = y?=w540:bool)
                  n526 = call-poly <vilib>:"Random Number (Range).vi"("lower bound (0)"=u64 0, "upper bound (100)"=u64 10) -> ("number"=w541:u64)  [unwired: 9 in]
                  n527 = Equal?(x=w542, y=2.0) -> (x = y?=w533:bool)
                  n528 = Equal?(x=w543, y=2.0) -> (x = y?=w534:bool)
                  n529 = Select(t=w536, s=w539, f=w533) -> (s? t:f=w530:bool)
                  n530 = Equal?(x=w526, y=w537) -> (x = y?=w538:bool)
                  n531 = Select(t=w535, s=w540, f=w534) -> (s? t:f=w531:bool)
                  n532 = Equal?(x=w541, y=2.0) -> (x = y?=w532:bool)
                  n533 = local write "Emergency Vehicle B"(w530) -> ()
                  n534 = local write "Emergency Vehicle A"(w531) -> ()
                  n535 = Select(t=w537, s=w538, f=w532) -> (s? t:f=w529:bool)
                  n536 = local write "Emergency Vehicle C"(w529) -> ()
                }
              }
            }
            n537 = local write "Lane 1y"(w489) -> ()
            n538 = local write "Lane 1r"(w489) -> ()
            n539 = local write "Lane 2g"(w489) -> ()
            n540 = local write "Lane 2y"(w489) -> ()
            n541 = local write "Lane 3g"(w489) -> ()
            n542 = local write "Lane 3y"(w489) -> ()
            n543 = local write "Lane 1g"(w490) -> ()
            n544 = local write "Lane 2r"(w490) -> ()
            n545 = local write "Lane 3r"(w490) -> ()
            n546 = local read "Lane 1g"() -> (w487:bool)
            n547 = local read "Emergency Vehicle A"() -> (w486:bool)
            n548 = case shown="True" w487 {
              frame False {
                n549 = local write "Car img A"(0.0 ("Car img A")) -> ()
              }
              frame True {
                n550 = while {
                  i -> [w513]
                  stop <- w512 stop-if-true
                  n551 = local read "Car img A"() -> (w511:dbl)
                  n552 = Not Equal?(x=w511, y=10.0) -> (x != y?=w505:bool)
                  n553 = Wait (ms)(milliseconds to wait=u32 100) -> ()  [unwired: 1 out]
                  n554 = local read "Timer"() -> (w508:dbl)
                  n555 = case shown="True" w505 {
                    frame False {
                      n556 = local write "Car img A"(0.0 ("Car img A")) -> ()
                    }
                    frame True {
                      n557 = local read "Car img A"() -> (w516:dbl)
                      n558 = Increment(x=w516) -> (x+1=w515:dbl)
                      n559 = local write "Car img A"(w515) -> ()
                    }
                  }
                  n560 = Multiply(x=w508, y=10.0) -> (x*y=w507:dbl)
                  n561 = Greater?(x=w513, y=w507) -> (0:w512:bool)
                }
              }
            }
            n562 = case shown="False" w486 {
              frame False {
                n563 = local write "EV img A"(0.0 ("EV img A")) -> ()
              }
              frame True {
                n564 = while {
                  i -> [w500]
                  stop <- w499 stop-if-true
                  n565 = local read "Cars A"() -> (w498:dbl)
                  n566 = Wait (ms)(milliseconds to wait=u32 100) -> ()  [unwired: 1 out]
                  n567 = Less?(x=w498, y=5.0) -> (x < y?=w497:bool)
                  n568 = case shown="True" w497 {
                    frame False {
                      n569 = local write "EV img A"(0.0 ("EV img A")) -> ()
                    }
                    frame True {
                      n570 = local read "EV img A"() -> (w503:dbl)
                      n571 = Increment(x=w503) -> (x+1=w502:dbl)
                      n572 = local write "EV img A"(w502) -> ()
                    }
                  }
                  n573 = local read "Timer"() -> (w494:dbl)
                  n574 = Multiply(x=w494, y=10.0) -> (x*y=w492:dbl)
                  n575 = Greater?(x=w500, y=w492) -> (0:w499:bool)
                }
              }
            }
            "Indicator" <- 1.0 ("Indicator")
          }
        }
      }
    }
  }
  "Timer" <- 9.0 ("Timer")
  "EV Num" <- 0.0 ("EV Num")
  "Emergency Lane" <- TRUE ("Emergency Lane")
  "EV Changer" <- 9.0 ("EV Changer")
  "EV Alert" <- FALSE ("EV Alert")
  "EV img A" <- 0.0 ("EV img A")
  "Car img B" <- 10.0 ("Car img B")
  "EV Img C" <- 10.0 ("EV Img C")
  "Car img  C" <- 10.0 ("Car img  C")
  "EV img b" <- 10.0 ("EV img b")
  "Car img A" <- 0.0 ("Car img A")
